vi "S4GUI.vi"() -> ()   [LabVIEW 2018] (continued)
                          tunnel: [w778 u32 13882323 u32 13882323] -> w773
                          tunnel: w775 -> [w777 _ _]
                          tunnel: w774 -> [w776 _ _]
                          frame Default {
                            n286 = case shown="True" w777 {
                              tunnel: [w779 w783] -> w778
                              tunnel: w776 -> [w779 w780]
                              frame False {
                              }
                              frame True {
                                n287 = Equal?(x=w780, y=u32 16776002) -> (x = y?=w782:bool)
                                n288 = case shown="False" w782 {
                                tunnel: [u32 16776002 u32 9346816] -> w783
                                frame False {
                                }
                                frame True {
                                }
                                }
                              }
                            }
                          }
                          frame "IDLE" {
                          }
                          frame "" {
                            # "sem resposta do ACS"
                          }
                        }
                      }
                    }
                    "Acq status string ch1" <- w701
                    n289 = case shown="True" w696 {
                      tunnel: w709 -> [_ w736]
                      tunnel: [u32 16739417 w738] -> w708
                      tunnel: w704 -> [_ w737]
                      tunnel: ["" ("CamStatus") w736] -> w698
                      frame False {
                      }
                      frame True {
                        n290 = property on="Acq status string ch3" class="Str"() -> ("Text.BGColor"=w739:u32)  [unwired: 2 in, 2 out]
                        n291 = case shown="Default" w736 {
                          tunnel: [w742 u32 13882323 u32 13882323] -> w738
                          tunnel: w737 -> [w741 _ _]
                          tunnel: w739 -> [w740 _ _]
                          frame Default {
                            n292 = case shown="True" w741 {
                              tunnel: [w743 w747] -> w742
                              tunnel: w740 -> [w743 w744]
                              frame False {
                              }
                              frame True {
                                n293 = Equal?(x=w744, y=u32 16776002) -> (x = y?=w746:bool)
                                n294 = case shown="True" w746 {
                                tunnel: [u32 16776002 u32 9346816] -> w747
                                frame False {
                                }
                                frame True {
                                }
                                }
                              }
                            }
                          }
                          frame "IDLE" {
                          }
                          frame "" {
                            # "sem resposta do ACS"
                          }
                        }
                      }
                    }
                    "Acq status string ch3" <- w698
                    n295 = case shown="True" w700 {
                      tunnel: w707 -> [_ w754]
                      tunnel: [u32 16739417 w756] -> w706
                      tunnel: w704 -> [_ w755]
                      tunnel: ["" ("CamStatus") w754] -> w699
                      frame False {
                      }
                      frame True {
                        n296 = property on="Acq status string ch2" class="Str"() -> ("Text.BGColor"=w757:u32)  [unwired: 2 in, 2 out]
                        n297 = case shown="\"IDLE\"" w754 {
                          tunnel: [w760 u32 13882323 u32 13882323] -> w756
                          tunnel: w755 -> [w759 _ _]
                          tunnel: w757 -> [w758 _ _]
                          frame Default {
                            n298 = case shown="False" w759 {
                              tunnel: [w761 w765] -> w760
                              tunnel: w758 -> [w761 w762]
                              frame False {
                              }
                              frame True {
                                n299 = Equal?(x=w762, y=u32 16776002) -> (x = y?=w764:bool)
                                n300 = case shown="True" w764 {
                                tunnel: [u32 16776002 u32 9346816] -> w765
                                frame False {
                                }
                                frame True {
                                }
                                }
                              }
                            }
                          }
                          frame "IDLE" {
                          }
                          frame "" {
                            # "sem resposta do ACS"
                          }
                        }
                      }
                    }
                    "Acq status string ch2" <- w699
                    n301 = property on="Acq status string ch2" class="Str"("Text.BGColor"=w706) -> ()  [unwired: 2 in, 2 out]
                    n302 = property on="Acq status string ch1" class="Str"("Text.BGColor"=w703) -> ()  [unwired: 2 in, 2 out]
                    n303 = property on="Acq status string ch3" class="Str"("Text.BGColor"=w708) -> ()  [unwired: 2 in, 2 out]
                    n304 = property on="Acq status string ch4" class="Str"("Text.BGColor"=w711) -> ()  [unwired: 2 in, 2 out]
                  }
                  frame #3 {
                    # "Atualiza status CANAL 1"
                    n305 = Unbundle By Name(w791) -> ("Frames done"=→"Exposure Done ch1":u32, "connection"=→"Channel 1" →"setupCH1":bool, "conf runing"=w788:bool)
                    n306 = property on="setupCH1" class="Bool (strict)"("Blinking"=w788) -> ()  [unwired: 2 in, 2 out]
                  }
                  frame #4 {
                    # "Atualiza status CANAL 2"
                    n307 = Unbundle By Name(w794) -> ("Frames done"=→"Exposure Done ch2":u32, "connection"=→"Channel 2" →"setupCH2":bool, "conf runing"=w792:bool)
                    n308 = property on="setupCH2" class="Bool (strict)"("Blinking"=w792) -> ()  [unwired: 2 in, 2 out]
                  }
                  frame #5 {
                    # "Atualiza status CANAL3"
                    n309 = Unbundle By Name(w798) -> ("Frames done"=→"Exposure Done ch3":u32, "connection"=→"Channel 3" →"setupCH3":bool, "conf runing"=w797:bool)
                    n310 = property on="setupCH3" class="Bool (strict)"("Blinking"=w797) -> ()  [unwired: 2 in, 2 out]
                  }
                  frame #6 {
                    # "Atualiza status CANAL4"
                    n311 = Unbundle By Name(w802) -> ("Frames done"=→"Exposure Done ch4":u32, "connection"=→"Channel 4" →"setupCH4":bool, "conf runing"=w801:bool)
                    n312 = property on="setupCH4" class="Bool (strict)"("Blinking"=w801) -> ()  [unwired: 2 in, 2 out]
                  }
                }
              }
              frame #9 {
                n313 = Unbundle By Name(w805) -> ("Instrument Status.mode"=w804:bool)
                n314 = case shown="True" w804 {
                  tunnel: [0 ("t") w819] -> w806
                  tunnel: w805 -> [_ w808]
                  frame False {
                    # "Fotometria: #PSD = 0"
                  }
                  frame True {
                    # "Polarimetria: calcula #PSD"
                    n315 = Unbundle By Name(w808) -> ("WPROT seq"=w812:u16)
                    n316 = Number To Boolean Array(number=w812) -> (Boolean array=w811:bool[])
                    n317 = for {
                      shift-right: [w823] -> w814
                      shift-left: 0 -> [w821]
                      tunnel: w811 -> [w820] mode=indexing
                      # "calcula qtd de 1s"
                      n318 = Increment(x=w821) -> (x+1=w822:i32)
                      n319 = Select(t=w822, s=w820, f=w821) -> (s? t:f=w823:i32)
                    }
                    n320 = property on="#Polarimetric Sequence Done" class="Slide (strict)"() -> ("Scale.Maximum"=w813:dbl)  [unwired: 2 in, 2 out]
                    n321 = To Long Integer(number=w813) -> (32bit integer=w815:i32)
                    n322 = Subtract(x=w815, y=w814) -> (x-y=w816:i32)
                    n323 = Decrement(x=w816) -> (x-1=w818:i32)
                    n324 = Less Than 0?(x=w818) -> (x < 0?=w817:bool)
                    n325 = Select(t=0, s=w817, f=w818) -> (s? t:f=w819:i32)
                  }
                }
                "#Polarimetric Sequence Done" <- w806
              }
              frame #10 {
                # "OVJ 2022-12-12: \nA visibilidade do Tab ObsEng sermpre \nacompanha a habilitação do tab4."
                n326 = Unbundle By Name(w828) -> ("Cluster ExpMode.tab4"=w825:T7, "Cluster Polarimetry"=w849:T15, "Cluster Mode Sync"=w859:T16)
                n327 = case shown="\"Disabled and Grayed Out\"" w825 {
                  tunnel: [TRUE ("Tabs Visible?") w861] -> w827
                  frame "Enabled", Default {
                  }
                  frame "Disabled and Grayed Out" {
                    n328 = disable-structure shown="Enabled" {
                      disable-tunnel: [TRUE ("Tabs Visible?") FALSE ("Tabs Visible?")] -> w861
                      frame Disabled {
                        # "DEBUG"
                      }
                      frame Enabled {
                      }
                    }
                  }
                }
                n329 = property on="Tab ObsEng" class="TabCtl (strict)"("Tabs Visible?"=w827) -> ()  [unwired: 2 in, 2 out]
                n330 = property on="Tab Acq Type" class="TabCtl (strict)"("DisabledEnum"=w825) -> (error out=w826:errorcluster)  [unwired: 2 in, 1 out]
                n331 = Unbundle By Name(w859) -> ("Start SM Text"=w858:string, "Star SM"=w857:T7, "Pause SM"=w856:T7, "Stop SM"=w855:T7, "Abort SM"=w854:T7, "#Index Cycles"=w853:T7, "#Cycles"=w852:T7, "SSM"=w851:T7, "Set SM"=w850:T7)
                n332 = property on="Observer" class="Str"(error in=w826, "DisabledEnum"=w825) -> (error out=w824:errorcluster)  [unwired: 1 in, 1 out]
                n333 = property on="Start SM" class="Bool"("BoolText.Text"=w858) -> ()  [unwired: 2 in, 2 out]
                n334 = property on="set keywords" class="Bool"(error in=w824, "DisabledEnum"=w825) -> ()  [unwired: 1 in, 2 out]
                n335 = property on="Start SM" class="Bool"("DisabledEnum"=w857) -> ()  [unwired: 2 in, 2 out]
                n336 = property on="Stop SM" class="Bool"("DisabledEnum"=w855) -> ()  [unwired: 2 in, 2 out]
                n337 = property on="Set SM" class="Bool"("DisabledEnum"=w850) -> ()  [unwired: 2 in, 2 out]
                n338 = property on="Pause SM" class="Bool"("DisabledEnum"=w856) -> ()  [unwired: 2 in, 2 out]
                n339 = property on="# Index Cycles" class="DigNum (strict)"("DisabledEnum"=w853) -> ()  [unwired: 2 in, 2 out]
                n340 = property on="# Cycles" class="DigNum (strict)"("DisabledEnum"=w852) -> ()  [unwired: 2 in, 2 out]
                n341 = property on="Abort SM" class="Bool"("DisabledEnum"=w854) -> ()  [unwired: 2 in, 2 out]
                n342 = property on="SSM" class="Ring (strict)"("DisabledEnum"=w851) -> ()  [unwired: 2 in, 2 out]
                n343 = Unbundle By Name(w849) -> ("Lambda Selector"=w848:T7, "Calibrator Selector"=w847:T7, "Set Waveplate"=w846:T7, "Select Positions"=w845:T7, "P0"=w844:T7, "P8"=w843:T7, "P1"=w842:T7, "P9"=w841:T7, "P2"=w840:T7, "P10"=w839:T7, "P3"=w838:T7, "P11"=w837:T7, "P4"=w836:T7, "P12"=w835:T7, "P5"=w834:T7, "P13"=w833:T7, "P6"=w832:T7, "P14"=w831:T7, "P7"=w830:T7, "P15"=w829:T7)
                n344 = property on="P0" class="Bool (strict)"("DisabledEnum"=w844) -> ()  [unwired: 2 in, 2 out]
                n345 = property on="Lambda Selector" class="Ring (strict)"("DisabledEnum"=w848) -> ()  [unwired: 2 in, 2 out]
                n346 = property on="Calibrator Selector" class="Ring (strict)"("DisabledEnum"=w847) -> ()  [unwired: 2 in, 2 out]
                n347 = property on="Set Waveplate" class="Bool"("DisabledEnum"=w846) -> ()  [unwired: 2 in, 2 out]
                n348 = property on="P1" class="Bool (strict)"("DisabledEnum"=w842) -> ()  [unwired: 2 in, 2 out]
                n349 = property on="P2" class="Bool (strict)"("DisabledEnum"=w840) -> ()  [unwired: 2 in, 2 out]
                n350 = property on="P3" class="Bool (strict)"("DisabledEnum"=w838) -> ()  [unwired: 2 in, 2 out]
                n351 = property on="P4" class="Bool (strict)"("DisabledEnum"=w836) -> ()  [unwired: 2 in, 2 out]
                n352 = property on="P5" class="Bool (strict)"("DisabledEnum"=w834) -> ()  [unwired: 2 in, 2 out]
                n353 = property on="P6" class="Bool (strict)"("DisabledEnum"=w832) -> ()  [unwired: 2 in, 2 out]
                n354 = property on="P7" class="Bool (strict)"("DisabledEnum"=w830) -> ()  [unwired: 2 in, 2 out]
                n355 = property on="Select Positions" class="Ring (strict)"("DisabledEnum"=w845) -> ()  [unwired: 2 in, 2 out]
                n356 = property on="P8" class="Bool (strict)"("DisabledEnum"=w843) -> ()  [unwired: 2 in, 2 out]
                n357 = property on="P15" class="Bool (strict)"("DisabledEnum"=w829) -> ()  [unwired: 2 in, 2 out]
                n358 = property on="P9" class="Bool (strict)"("DisabledEnum"=w841) -> ()  [unwired: 2 in, 2 out]
                n359 = property on="P10" class="Bool (strict)"("DisabledEnum"=w839) -> ()  [unwired: 2 in, 2 out]
                n360 = property on="P11" class="Bool (strict)"("DisabledEnum"=w837) -> ()  [unwired: 2 in, 2 out]
                n361 = property on="P12" class="Bool (strict)"("DisabledEnum"=w835) -> ()  [unwired: 2 in, 2 out]
                n362 = property on="P13" class="Bool (strict)"("DisabledEnum"=w833) -> ()  [unwired: 2 in, 2 out]
                n363 = property on="P14" class="Bool (strict)"("DisabledEnum"=w831) -> ()  [unwired: 2 in, 2 out]
              }
              frame #11 {
                n364 = Unbundle By Name(w875) -> ("Cluster Mode CH1"=w874:T17)
                n365 = Unbundle By Name(w874) -> ("Start ch1 Text"=w873:string, "#cycles ch1"=w872:T7, "Start ch1"=w871:T7, "Pause ch1"=w870:T7, "Abort ch1"=w869:T7, "Stop ch1"=w868:T7, "Exptime ch1"=w867:T7, "Exp ch1"=w866:T7, "Set Cooler"=w865:T7, "Set Temp"=w864:T7)
                n366 = property on="Start ch1" class="Bool"("BoolText.Text"=w873) -> ()  [unwired: 2 in, 2 out]
                n367 = property on="Abort ch1" class="Bool"("DisabledEnum"=w869) -> ()  [unwired: 2 in, 2 out]
                n368 = property on="Stop ch1" class="Bool"("DisabledEnum"=w868) -> ()  [unwired: 2 in, 2 out]
                n369 = property on="#cycles ch1" class="DigNum (strict)"("DisabledEnum"=w872) -> ()  [unwired: 2 in, 2 out]
                n370 = property on="Cooler 1" class="Bool (strict)"("DisabledEnum"=w865) -> ()  [unwired: 2 in, 2 out]
                n371 = property on="Exptime ch1" class="DigNum (strict)"("DisabledEnum"=w867) -> ()  [unwired: 2 in, 2 out]
                n372 = property on="Start ch1" class="Bool"("DisabledEnum"=w871) -> ()  [unwired: 2 in, 2 out]
                n373 = property on="Set Temp 1" class="Bool"("DisabledEnum"=w864) -> ()  [unwired: 2 in, 2 out]
                n374 = property on="Exp ch1" class="DigNum (strict)"("DisabledEnum"=w866) -> ()  [unwired: 2 in, 2 out]
                n375 = property on="Pause ch1" class="Bool"("DisabledEnum"=w870) -> ()  [unwired: 2 in, 2 out]
              }
              frame #12 {
                n376 = Unbundle By Name(w887) -> ("Cluster Mode CH2"=w886:T18)
                n377 = Unbundle By Name(w886) -> ("Start ch2 Text"=w885:string, "#cycles ch2"=w884:T7, "Start ch2"=w883:T7, "Pause ch2"=w882:T7, "Stop ch2"=w881:T7, "Abort ch2"=w880:T7, "Exptime ch2"=w879:T7, "Exp ch2"=w878:T7, "Set Cooler"=w877:T7, "Set Temp"=w876:T7)
                n378 = property on="Start ch2" class="Bool"("BoolText.Text"=w885) -> ()  [unwired: 2 in, 2 out]
                n379 = property on="Stop ch2" class="Bool"("DisabledEnum"=w881) -> ()  [unwired: 2 in, 2 out]
                n380 = property on="Abort ch2" class="Bool"("DisabledEnum"=w880) -> ()  [unwired: 2 in, 2 out]
                n381 = property on="Cooler 2" class="Bool (strict)"("DisabledEnum"=w877) -> ()  [unwired: 2 in, 2 out]
                n382 = property on="#cycles ch2" class="DigNum (strict)"("DisabledEnum"=w884) -> ()  [unwired: 2 in, 2 out]
                n383 = property on="Exptime ch2" class="DigNum (strict)"("DisabledEnum"=w879) -> ()  [unwired: 2 in, 2 out]
                n384 = property on="Set Temp 2" class="Bool"("DisabledEnum"=w876) -> ()  [unwired: 2 in, 2 out]
                n385 = property on="Start ch2" class="Bool"("DisabledEnum"=w883) -> ()  [unwired: 2 in, 2 out]
                n386 = property on="Exp ch2" class="DigNum (strict)"("DisabledEnum"=w878) -> ()  [unwired: 2 in, 2 out]
                n387 = property on="Pause ch2" class="Bool"("DisabledEnum"=w882) -> ()  [unwired: 2 in, 2 out]
              }
              frame #13 {
                n388 = Unbundle By Name(w899) -> ("Cluster Mode CH3"=w898:T19)
                n389 = Unbundle By Name(w898) -> ("Start ch3 Text"=w897:string, "#cycles ch3"=w896:T7, "Start ch3"=w895:T7, "Pause ch3"=w894:T7, "Stop ch3"=w893:T7, "Abort ch3"=w892:T7, "Exptime ch3"=w891:T7, "Exp ch3"=w890:T7, "Set Cooler"=w889:T7, "Set Temp"=w888:T7)
                n390 = property on="Start ch3" class="Bool"("BoolText.Text"=w897) -> ()  [unwired: 2 in, 2 out]
                n391 = property on="Stop ch3" class="Bool"("DisabledEnum"=w893) -> ()  [unwired: 2 in, 2 out]
                n392 = property on="Abort ch3" class="Bool"("DisabledEnum"=w892) -> ()  [unwired: 2 in, 2 out]
                n393 = property on="Cooler 3" class="Bool (strict)"("DisabledEnum"=w889) -> ()  [unwired: 2 in, 2 out]
                n394 = property on="#cycles ch3" class="DigNum (strict)"("DisabledEnum"=w896) -> ()  [unwired: 2 in, 2 out]
                n395 = property on="Set Temp 3" class="Bool"("DisabledEnum"=w888) -> ()  [unwired: 2 in, 2 out]
                n396 = property on="Exptime ch3" class="DigNum (strict)"("DisabledEnum"=w891) -> ()  [unwired: 2 in, 2 out]
                n397 = property on="Start ch3" class="Bool"("DisabledEnum"=w895) -> ()  [unwired: 2 in, 2 out]
                n398 = property on="Exp ch3" class="DigNum (strict)"("DisabledEnum"=w890) -> ()  [unwired: 2 in, 2 out]
                n399 = property on="Pause ch3" class="Bool"("DisabledEnum"=w894) -> ()  [unwired: 2 in, 2 out]
              }
              frame #14 {
                n400 = Unbundle By Name(w911) -> ("Cluster Mode CH4"=w910:T20)
                n401 = Unbundle By Name(w910) -> ("Start ch4 Text"=w909:string, "#cycles ch4"=w908:T7, "Start ch4"=w907:T7, "Pause ch4"=w906:T7, "Stop ch4"=w905:T7, "Abort ch4"=w904:T7, "Exptime ch4"=w903:T7, "Exp ch4"=w902:T7, "Set Cooler"=w901:T7, "Set Temp"=w900:T7)
                n402 = property on="Start ch4" class="Bool"("BoolText.Text"=w909) -> ()  [unwired: 2 in, 2 out]
                n403 = property on="Stop ch4" class="Bool"("DisabledEnum"=w905) -> ()  [unwired: 2 in, 2 out]
                n404 = property on="Cooler 4" class="Bool (strict)"("DisabledEnum"=w901) -> ()  [unwired: 2 in, 2 out]
                n405 = property on="Set Temp 4" class="Bool"("DisabledEnum"=w900) -> ()  [unwired: 2 in, 2 out]
                n406 = property on="Abort ch4" class="Bool"("DisabledEnum"=w904) -> ()  [unwired: 2 in, 2 out]
                n407 = property on="#cycles ch4" class="DigNum (strict)"("DisabledEnum"=w908) -> ()  [unwired: 2 in, 2 out]
                n408 = property on="Exptime ch4" class="DigNum (strict)"("DisabledEnum"=w903) -> ()  [unwired: 2 in, 2 out]
                n409 = property on="Start ch4" class="Bool"("DisabledEnum"=w907) -> ()  [unwired: 2 in, 2 out]
                n410 = property on="Exp ch4" class="DigNum (strict)"("DisabledEnum"=w902) -> ()  [unwired: 2 in, 2 out]
                n411 = property on="Pause ch4" class="Bool"("DisabledEnum"=w906) -> ()  [unwired: 2 in, 2 out]
              }
              frame #15 {
                # "Carrega coluna do Channel 1"
                # "Aba:  Eng->Camera"
                n412 = Unbundle By Name(w995) -> ("ChannelA_CCD"=w919:T21, "CHA_Checked Params"=w986:T22, "ChannelA_Status.connection"=w918:bool)
                n413 = Unbundle By Name(w986) -> ("ACQUISITION_MODE"=w943:bool, "TRIGGER_MODE"=w944:bool, "READ_MODE"=w945:bool, "PREAMP"=w953:bool, "READOUT_RATE"=w954:bool, "VERTICAL_SHIFT_SPEED"=w955:bool, "EM_MODE"=w956:bool, "EM_GAIN"=w946:bool, "SHUTTER_MODE"=w947:bool, "SHUTTER_TTL"=w948:bool, "SHUTTER_OPENING_TIME"=w949:bool, "SHUTTER_CLOSING_TIME"=w950:bool, "VBIN"=w951:bool, "HBIN"=w952:bool, "INITIAL_LINE"=w964:bool, "INITIAL_COLUMN"=w980:bool, "FINAL_LINE"=w985:bool, "FINAL_COLUMN"=w978:bool, "FRAME_TRANSFER"=w974:bool, "VERTICAL_CLOCK_VOLTAGE"=w973:bool, "AD_CHANNEL"=w972:bool)
                n414 = Unbundle By Name(w919) -> ("INITIAL_LINE"=w941:u16, "INITIAL_COLUMN"=w940:u16, "FINAL_LINE"=w939:u16, "FINAL_COLUMN"=w938:u16, "VBIN"=w937:u16, "HBIN"=w936:u16, "PREAMP"=w935:u8, "EM_GAIN"=w934:u16, "READOUT_RATE"=w933:u8, "SHUTTER_OPENNING_TIME"=w932:u16, "SHUTTER_CLOSING_TIME"=w931:u16, "VERTICAL_SHIFT_SPEED"=w930:u8, "READ_MODE"=w929:u8, "VERTICAL_CLOCK_VOLTAGE"=w928:u8, "AD_CHANNEL"=w927:u32, "SHUTTER_MODE"=w926:u8, "SHUTTER_TTL"=w925:u8, "TRIGGER_MODE"=w924:u8, "FRAME_TRANSFER"=w923:bool, "ACQUISITION_MODE"=w921:u8, "EM_MODE"=w920:u8)
                n415 = Equal?(x=w990, y="none") -> (x = y?=w987:bool)
                n416 = Equal?(x=w990, y="default.cfg") -> (x = y?=w988:bool)
                n417 = Or(x=w988, y=w987) -> (x .or. y?=w989:bool)
                n418 = case shown="True" w989 {
                  tunnel: [T7."Enabled" ("Disabled") T7."Disabled and Grayed Out" ("Disabled")] -> w992
                  frame False {
                    # "Se Curr Conf File != default.cfg,\nhabilita botão de Salvar."
                  }
                  frame True {
                    # "Não é permitido salvar em \ncima de default.cfg"
                  }
                }
                n419 = case shown="True" w918 {
                  tunnel: w919 -> [_ w1003]
                  tunnel: [w996 w1002] -> w917
                  tunnel: [w996 w1001] -> w916
                  tunnel: [w996 w1000] -> w915
                  tunnel: [w996 w999] -> w914
                  tunnel: [w996 w998] -> w913
                  tunnel: [w996 w997] -> w912
                  frame False {
                    w996 = "" ("RO1")
                  }
                  frame True {
                    n420 = stacked-sequence "Atualizacao dos indicadores inferiores do CANAL A da tela principal" {
                      tunnel: w1003 -> [w1018 w1021 w1026 w1035 w1038 w1042]
                      tunnel: [w1004 _ _ _ _ _] -> w1002
                      tunnel: [_ w1019 _ _ _ _] -> w1001
                      tunnel: [_ _ w1024 _ _ _] -> w1000
                      tunnel: [_ _ _ w1029 _ _] -> w999
                      tunnel: [_ _ _ _ w1036 _] -> w998
                      tunnel: [_ _ _ _ _ w1039] -> w997
                      frame #0 {
                        # "SubImage"
                        n421 = Unbundle By Name(w1018) -> ("INITIAL_LINE"=w1016:u16, "FINAL_LINE"=w1015:u16, "INITIAL_COLUMN"=w1014:u16, "FINAL_COLUMN"=w1013:u16)
                        n422 = Number To Decimal String(number=w1016) -> (decimal integer string=w1012:string)  [unwired: 1 in]
                        n423 = Number To Decimal String(number=w1015) -> (decimal integer string=w1010:string)  [unwired: 1 in]
                        n424 = Number To Decimal String(number=w1014) -> (decimal integer string=w1008:string)  [unwired: 1 in]
                        n425 = Number To Decimal String(number=w1013) -> (decimal integer string=w1006:string)  [unwired: 1 in]
                        n426 = Concatenate Strings("[", w1012, ":", w1010, ",", w1008, ":", w1006, "]") -> (w1004:string)
                      }
                      frame #1 {
                        # "Em Active"
                        n427 = Unbundle By Name(w1021) -> ("EM_MODE"=w1020:u8)
                        n428 = case shown="0, Default" w1020 {
                          tunnel: ["Electron M." ("EmActive1") "Convent." ("EmActive1")] -> w1019
                          frame 0, Default {
                          }
                          frame 1 {
                          }
                        }
                      }
                      frame #2 {
                        # "Pre Amp"
                        n429 = Unbundle By Name(w1026) -> ("PREAMP"=w1025:u8)
                        n430 = case shown="1" w1025 {
                          tunnel: ["Gain 1" ("EmActive1") "Gain 2" ("EmActive1")] -> w1024
                          frame 0, Default {
                          }
                          frame 1 {
                          }
                        }
                      }
                      frame #3 {
                        # "Binning"
                        n431 = Unbundle By Name(w1035) -> ("VBIN"=w1034:u16, "HBIN"=w1033:u16)
                        n432 = Number To Decimal String(number=w1033) -> (decimal integer string=w1030:string)  [unwired: 1 in]
                        n433 = Number To Decimal String(number=w1034) -> (decimal integer string=w1032:string)  [unwired: 1 in]
                        n434 = Concatenate Strings(w1032, "x", w1030) -> (w1029:string)
                      }
                      frame #4 {
                        # "Gain"
                        n435 = Unbundle By Name(w1038) -> ("EM_GAIN"=w1037:u16)
                        n436 = Number To Decimal String(number=w1037) -> (decimal integer string=w1036:string)  [unwired: 1 in]
                      }
                      frame #5 {
                        # "Readout"
                        n437 = Unbundle By Name(w1042) -> ("EM_MODE"=w1041:u8, "READOUT_RATE"=w1040:u8)
                        n438 = case shown="1" w1041 {
                          tunnel: w1040 -> [w1044 w1050]
                          tunnel: [w1043 w1049] -> w1039
                          frame 0, Default {
                            n439 = case shown="3" w1044 {
                              tunnel: ["30 MHz" ("EmActive1") "20 MHz" ("EmActive1") "10 MHz" ("EmActive1") "1 MHz" ("EmActive1")] -> w1043
                              frame 0, Default {
                              }
                              frame 1 {
                              }
                              frame 2 {
                              }
                              frame 3 {
                              }
                            }
                          }
                          frame 1 {
                            n440 = case shown="1" w1050 {
                              tunnel: ["1 MHz" ("EmActive1") "0.1 MHz" ("EmActive1")] -> w1049
                              frame 0, Default {
                              }
                              frame 1 {
                              }
                            }
                          }
                        }
                      }
                    }
                  }
                }
                n441 = Not(x=w978) -> (.not. x?=w979:bool)
                n442 = Not(x=w974) -> (.not. x?=w976:bool)
                n443 = Not(x=w973) -> (.not. x?=w977:bool)
                n444 = Not(x=w972) -> (.not. x?=w975:bool)
                n445 = Not(x=w964) -> (.not. x?=w982:bool)
                n446 = Not(x=w980) -> (.not. x?=w981:bool)
                n447 = Not(x=w985) -> (.not. x?=w984:bool)
                n448 = property on="Image FInal Column" class="DigNum (strict)"("Blinking"=w979) -> ()  [unwired: 2 in, 2 out]
                n449 = property on="Frame Transfer" class="Bool (strict)"("Blinking"=w976) -> ()  [unwired: 2 in, 2 out]
                n450 = property on="Vertical Clock Voltage" class="Ring (strict)"("Blinking"=w977) -> ()  [unwired: 2 in, 2 out]
                n451 = property on="A/D  Channel" class="DigNum (strict)"("Blinking"=w975) -> ()  [unwired: 2 in, 2 out]
                n452 = property on="Image Initial Line" class="DigNum (strict)"("Blinking"=w982) -> ()  [unwired: 2 in, 2 out]
                n453 = property on="Image Initial Column" class="DigNum (strict)"("Blinking"=w981) -> ()  [unwired: 2 in, 2 out]
                n454 = property on="Image Final Line" class="DigNum (strict)"("Blinking"=w984) -> ()  [unwired: 2 in, 2 out]
                n455 = property on="Save Button" class="Bool (strict)"("DisabledEnum"=w992) -> ()  [unwired: 2 in, 2 out]
                n456 = Not(x=w949) -> (.not. x?=w968:bool)
                n457 = Not(x=w950) -> (.not. x?=w970:bool)
                n458 = Not(x=w951) -> (.not. x?=w969:bool)
                n459 = Not(x=w952) -> (.not. x?=w971:bool)
                n460 = Not(x=w946) -> (.not. x?=w966:bool)
                n461 = Not(x=w947) -> (.not. x?=w967:bool)
                n462 = Not(x=w948) -> (.not. x?=w965:bool)
                n463 = property on="Shutter Openning Time" class="DigNum (strict)"("Blinking"=w968) -> ()  [unwired: 2 in, 2 out]
                n464 = property on="Shutter Closing Time" class="DigNum (strict)"("Blinking"=w970) -> ()  [unwired: 2 in, 2 out]
                n465 = property on="Vertical Binning" class="DigNum (strict)"("Blinking"=w969) -> ()  [unwired: 2 in, 2 out]
                n466 = property on="Horizontal Binning" class="DigNum (strict)"("Blinking"=w971) -> ()  [unwired: 2 in, 2 out]
                n467 = property on="CCD EM Gain" class="DigNum (strict)"("Blinking"=w966) -> ()  [unwired: 2 in, 2 out]
                n468 = property on="Shutter Mode" class="Ring (strict)"("Blinking"=w967) -> ()  [unwired: 2 in, 2 out]
                n469 = property on="Shutter TTL" class="Ring (strict)"("Blinking"=w965) -> ()  [unwired: 2 in, 2 out]
                n470 = First Call?() -> (First Call?: T/F=w942:bool)
                n471 = case shown="True" w942 {
                  tunnel: w941 -> [_ w1073]
                  tunnel: w940 -> [_ w1072]
                  tunnel: w939 -> [_ w1071]
                  tunnel: w938 -> [_ w1070]
                  tunnel: w937 -> [_ w1069]
                  tunnel: w936 -> [_ w1068]
                  tunnel: w935 -> [_ w1067]
                  tunnel: w934 -> [_ w1066]
                  tunnel: w933 -> [_ w1065]
                  tunnel: w932 -> [_ w1064]
                  tunnel: w931 -> [_ w1063]
                  tunnel: w930 -> [_ w1062]
                  tunnel: w929 -> [_ w1061]
                  tunnel: w928 -> [_ w1060]
                  tunnel: w927 -> [_ w1059]
                  tunnel: w926 -> [_ w1058]
                  tunnel: w925 -> [_ w1057]
                  tunnel: w924 -> [_ w1056]
                  tunnel: w923 -> [_ w1055]
                  tunnel: w921 -> [_ w1054]
                  tunnel: w920 -> [_ w1053]
                  frame False {
                  }
                  frame True {
                    n472 = local read "Input Cluster"() -> (w1077:T5)
                    n473 = Unbundle By Name(w1077) -> ("Parameters"=w1075:T23)
                    n474 = Bundle By Name(cluster=w1075, "Image \nInitial Line"=w1073, "Image\nInitial Column"=w1072, "Image\nFinal Line"=w1071, "Image\nFInal Column"=w1070, "Vertical\nBinning"=w1069, "Horizontal\nBinning"=w1068, "Pre-amplification\nGain"=w1067, "CCD\nEM Gain"=w1066, "Readout\nRate"=w1065, "Shutter\nOpenning Time"=w1064, "Shutter\nClosing Time"=w1063, "Vertical\nShift Speed"=w1062, "Read\nMode"=w1061, "Vertical\nClock Voltage"=w1060, "A/D \nChannel"=w1059, "Shutter\nMode"=w1058, "Shutter\nTTL"=w1057, "Trigger\nMode"=w1056, "Frame\nTransfer"=w1055, "Acquisition\nMode"=w1054, "CCD \nEM Mode"=w1053) -> (w1074:T23)
                    n475 = Bundle By Name(cluster=w1077, "Parameters"=w1074) -> (w1076:T5)
                    n476 = local write "Input Cluster"(w1076) -> ()
                  }
                }
                n477 = Not(x=w943) -> (.not. x?=w957:bool)
                n478 = local read "Cameras Cluster"() -> (w994:T6)
                n479 = Bundle By Name(cluster=w994, "Current Configuration.Image Initial Line"=w941, "Current Configuration.Image Initial Column"=w940, "Current Configuration.Image Final Line"=w939, "Current Configuration.Image FInal Column"=w938, "Current Configuration.Vertical Binning"=w937, "Current Configuration.Horizontal Binning"=w936, "Current Configuration.Pre-amplification Gain"=w935, "Current Configuration.CCD EM Gain"=w934, "Current Configuration.Readout Rate"=w933, "Current Configuration.Shutter Openning Time"=w932, "Current Configuration.Shutter Closing Time"=w931, "Current Configuration.Vertical Shift Speed"=w930, "Current Configuration.Read Mode"=w929, "Current Configuration.Vertical Clock Voltage"=w928, "Current Configuration.A/D  Channel"=w927, "Current Configuration.Shutter Mode"=w926, "Current Configuration.Shutter TTL"=w925, "Current Configuration.Trigger Mode"=w924, "Current Configuration.Frame Transfer"=w923, "Current Configuration.Acquisition Mode"=w921, "Current Configuration.CCD EM Mode"=w920) -> (w922:T6)
                n480 = Not(x=w954) -> (.not. x?=w960:bool)
                n481 = Not(x=w955) -> (.not. x?=w958:bool)
                n482 = Not(x=w956) -> (.not. x?=w959:bool)
                n483 = Not(x=w944) -> (.not. x?=w962:bool)
                n484 = Not(x=w945) -> (.not. x?=w961:bool)
                n485 = Not(x=w953) -> (.not. x?=w963:bool)
                n486 = local write "RO1"(w912) -> ()
                n487 = local write "SI1"(w917) -> ()
                n488 = local write "EA1"(w916) -> ()
                n489 = local write "PA1"(w915) -> ()
                n490 = local write "B1"(w914) -> ()
                n491 = local write "G1"(w913) -> ()
                n492 = property on="Acquisition Mode" class="Ring (strict)"("Blinking"=w957) -> ()  [unwired: 2 in, 2 out]
                n493 = property on="Readout Rate" class="Ring (strict)"("Blinking"=w960) -> ()  [unwired: 2 in, 2 out]
                n494 = property on="Vertical Shift Speed" class="Ring (strict)"("Blinking"=w958) -> ()  [unwired: 2 in, 2 out]
                n495 = property on="CCD EM Mode" class="Ring (strict)"("Blinking"=w959) -> ()  [unwired: 2 in, 2 out]
                n496 = property on="Trigger Mode" class="Ring (strict)"("Blinking"=w962) -> ()  [unwired: 2 in, 2 out]
                n497 = property on="Read Mode" class="Ring (strict)"("Blinking"=w961) -> ()  [unwired: 2 in, 2 out]
                n498 = property on="Pre-amplification Gain" class="Ring (strict)"("Blinking"=w963) -> ()  [unwired: 2 in, 2 out]
                n499 = local write "Cameras Cluster"(w922) -> ()
                n500 = Compound Arithmetic op=AND(w943, w944, w945, w953, w954, w955, w956, w946, w947, w948, w949, w950, w951, w952, w964, w980, w985, w978, w974, w973, w972) -> (→"CCD checked 1":bool)
                "Current Configuration File:" <- w990
              }
              frame #16 {
                # "Carrega coluna do Channel 2"
                # "Aba:  Eng->Camera"
                n501 = Unbundle By Name(w1155) -> ("ChannelB_CCD"=w1087:T21, "CHB_Checked Params"=w1088:T22, "ChannelB_Status.connection"=w1086:bool)
                n502 = Unbundle By Name(w1088) -> ("ACQUISITION_MODE"=w1106:bool, "TRIGGER_MODE"=w1105:bool, "READ_MODE"=w1104:bool, "PREAMP"=w1103:bool, "READOUT_RATE"=w1102:bool, "VERTICAL_SHIFT_SPEED"=w1101:bool, "EM_MODE"=w1100:bool, "EM_GAIN"=w1113:bool, "SHUTTER_MODE"=w1112:bool, "SHUTTER_TTL"=w1111:bool, "SHUTTER_OPENING_TIME"=w1110:bool, "SHUTTER_CLOSING_TIME"=w1109:bool, "VBIN"=w1108:bool, "HBIN"=w1107:bool, "INITIAL_LINE"=w1120:bool, "INITIAL_COLUMN"=w1119:bool, "FINAL_LINE"=w1118:bool, "FINAL_COLUMN"=w1117:bool, "FRAME_TRANSFER"=w1116:bool, "VERTICAL_CLOCK_VOLTAGE"=w1115:bool, "AD_CHANNEL"=w1114:bool)
                n503 = case shown="True" w1086 {
                  tunnel: w1087 -> [_ w1163]
                  tunnel: [w1156 w1162] -> w1085
                  tunnel: [w1156 w1161] -> w1084
                  tunnel: [w1156 w1160] -> w1083
                  tunnel: [w1156 w1159] -> w1082
                  tunnel: [w1156 w1158] -> w1081
                  tunnel: [w1156 w1157] -> w1080
                  frame False {
                    w1156 = "" ("EmActive1")
                  }
                  frame True {
                    n504 = stacked-sequence "Atualizacao dos indicadores inferiores do CANAL B da tela principal" {
                      tunnel: w1163 -> [w1178 w1181 w1186 w1195 w1198 w1202]
                      tunnel: [_ w1179 _ _ _ _] -> w1162
                      tunnel: [_ _ w1184 _ _ _] -> w1161
                      tunnel: [_ _ _ w1189 _ _] -> w1160
                      tunnel: [_ _ _ _ w1196 _] -> w1159
                      tunnel: [_ _ _ _ _ w1199] -> w1158
                      tunnel: [w1164 _ _ _ _ _] -> w1157
                      frame #0 {
                        # "SubImage"
                        n505 = Unbundle By Name(w1178) -> ("INITIAL_LINE"=w1176:u16, "FINAL_LINE"=w1175:u16, "INITIAL_COLUMN"=w1174:u16, "FINAL_COLUMN"=w1173:u16)
                        n506 = Number To Decimal String(number=w1176) -> (decimal integer string=w1172:string)  [unwired: 1 in]
                        n507 = Number To Decimal String(number=w1175) -> (decimal integer string=w1170:string)  [unwired: 1 in]
                        n508 = Number To Decimal String(number=w1174) -> (decimal integer string=w1168:string)  [unwired: 1 in]
                        n509 = Number To Decimal String(number=w1173) -> (decimal integer string=w1166:string)  [unwired: 1 in]
                        n510 = Concatenate Strings("[", w1172, ":", w1170, ",", w1168, ":", w1166, "]") -> (w1164:string)
                      }
                      frame #1 {
                        # "Em Active"
                        n511 = Unbundle By Name(w1181) -> ("EM_MODE"=w1180:u8)
                        n512 = case shown="0, Default" w1180 {
                          tunnel: ["Electron M." ("EmActive1") "Convent." ("EmActive1")] -> w1179
                          frame 0, Default {
                          }
                          frame 1 {
                          }
                        }
                      }
                      frame #2 {
                        # "Pre Amp"
                        n513 = Unbundle By Name(w1186) -> ("PREAMP"=w1185:u8)
                        n514 = case shown="1" w1185 {
                          tunnel: ["Gain 1" ("EmActive1") "Gain 2" ("EmActive1")] -> w1184
                          frame 0, Default {
                          }
                          frame 1 {
                          }
                        }
                      }
                      frame #3 {
                        # "Binning"
                        n515 = Unbundle By Name(w1195) -> ("VBIN"=w1194:u16, "HBIN"=w1193:u16)
                        n516 = Number To Decimal String(number=w1193) -> (decimal integer string=w1191:string)  [unwired: 1 in]
                        n517 = Number To Decimal String(number=w1194) -> (decimal integer string=w1192:string)  [unwired: 1 in]
                        n518 = Concatenate Strings(w1192, "x", w1191) -> (w1189:string)
                      }
                      frame #4 {
                        # "Gain"
                        n519 = Unbundle By Name(w1198) -> ("EM_GAIN"=w1197:u16)
                        n520 = Number To Decimal String(number=w1197) -> (decimal integer string=w1196:string)  [unwired: 1 in]
                      }
                      frame #5 {
                        # "Readout"
                        n521 = Unbundle By Name(w1202) -> ("EM_MODE"=w1201:u8, "READOUT_RATE"=w1200:u8)
                        n522 = case shown="0, Default" w1201 {
                          tunnel: w1200 -> [w1204 w1210]
                          tunnel: [w1203 w1209] -> w1199
                          frame 0, Default {
                            n523 = case shown="0, Default" w1204 {
                              tunnel: ["30 MHz" ("EmActive1") "20 MHz" ("EmActive1") "10 MHz" ("EmActive1") "1 MHz" ("EmActive1")] -> w1203
                              frame 0, Default {
                              }
                              frame 1 {
                              }
                              frame 2 {
                              }
                              frame 3 {
                              }
                            }
                          }
                          frame 1 {
                            n524 = case shown="1" w1210 {
                              tunnel: ["1 MHz" ("EmActive1") "0.1 MHz" ("EmActive1")] -> w1209
                              frame 0, Default {
                              }
                              frame 1 {
                              }
                            }
                          }
                        }
                      }
                    }
                  }
                }
                n525 = Unbundle By Name(w1087) -> ("INITIAL_LINE"=w1093:u16, "INITIAL_COLUMN"=w1091:u16, "FINAL_LINE"=w1094:u16, "FINAL_COLUMN"=w1092:u16, "VBIN"=w1097:u16, "HBIN"=w1152:u16, "PREAMP"=w1096:u8, "EM_GAIN"=w1095:u16, "READOUT_RATE"=w1090:u8, "SHUTTER_OPENNING_TIME"=w1151:u16, "SHUTTER_CLOSING_TIME"=w1150:u16, "VERTICAL_SHIFT_SPEED"=w1149:u8, "READ_MODE"=w1148:u8, "VERTICAL_CLOCK_VOLTAGE"=w1147:u8, "AD_CHANNEL"=w1146:u32, "SHUTTER_MODE"=w1143:u8, "SHUTTER_TTL"=w1144:u8, "TRIGGER_MODE"=w1098:u8, "FRAME_TRANSFER"=w1099:bool, "ACQUISITION_MODE"=w1145:u8, "EM_MODE"=w1089:u8)
                n526 = Not(x=w1117) -> (.not. x?=w1138:bool)
                n527 = Not(x=w1116) -> (.not. x?=w1136:bool)
                n528 = Not(x=w1115) -> (.not. x?=w1137:bool)
                n529 = Not(x=w1114) -> (.not. x?=w1135:bool)
                n530 = Not(x=w1120) -> (.not. x?=w1140:bool)
                n531 = Not(x=w1119) -> (.not. x?=w1139:bool)
                n532 = Not(x=w1118) -> (.not. x?=w1141:bool)
                n533 = property on="Image FInal Column 2" class="DigNum (strict)"("Blinking"=w1138) -> ()  [unwired: 2 in, 2 out]
                n534 = property on="Frame Transfer 2" class="Bool (strict)"("Blinking"=w1136) -> ()  [unwired: 2 in, 2 out]
                n535 = property on="Vertical Clock Voltage 2" class="Ring (strict)"("Blinking"=w1137) -> ()  [unwired: 2 in, 2 out]
                n536 = property on="A/D Channel 2" class="DigNum (strict)"("Blinking"=w1135) -> ()  [unwired: 2 in, 2 out]
                n537 = property on="Image Initial Line 2" class="DigNum (strict)"("Blinking"=w1140) -> ()  [unwired: 2 in, 2 out]
                n538 = property on="Image Initial Column 2" class="DigNum (strict)"("Blinking"=w1139) -> ()  [unwired: 2 in, 2 out]
                n539 = property on="Image Final Line 2" class="DigNum (strict)"("Blinking"=w1141) -> ()  [unwired: 2 in, 2 out]
                n540 = Not(x=w1110) -> (.not. x?=w1131:bool)
                n541 = Not(x=w1109) -> (.not. x?=w1133:bool)
                n542 = Not(x=w1108) -> (.not. x?=w1132:bool)
                n543 = Not(x=w1107) -> (.not. x?=w1134:bool)
                n544 = Not(x=w1113) -> (.not. x?=w1129:bool)
                n545 = Not(x=w1112) -> (.not. x?=w1130:bool)
                n546 = Not(x=w1111) -> (.not. x?=w1128:bool)
                n547 = property on="Shutter Openning Time 2" class="DigNum (strict)"("Blinking"=w1131) -> ()  [unwired: 2 in, 2 out]
                n548 = property on="Shutter Closing Time 2" class="DigNum (strict)"("Blinking"=w1133) -> ()  [unwired: 2 in, 2 out]
                n549 = property on="Vertical Binning 2" class="DigNum (strict)"("Blinking"=w1132) -> ()  [unwired: 2 in, 2 out]
                n550 = property on="Horizontal Binning 2" class="DigNum (strict)"("Blinking"=w1134) -> ()  [unwired: 2 in, 2 out]
                n551 = property on="CCD EM Gain 2" class="DigNum (strict)"("Blinking"=w1129) -> ()  [unwired: 2 in, 2 out]
                n552 = property on="Shutter Mode 2" class="Ring (strict)"("Blinking"=w1130) -> ()  [unwired: 2 in, 2 out]
                n553 = property on="Shutter TTL 2" class="Ring (strict)"("Blinking"=w1128) -> ()  [unwired: 2 in, 2 out]
                n554 = local read "Cameras Cluster"() -> (w1154:T6)
                n555 = Bundle By Name(cluster=w1154, "Current Configuration.Image Initial Line 2"=w1093, "Current Configuration.Image Initial Column 2"=w1091, "Current Configuration.Image Final Line 2"=w1094, "Current Configuration.Image FInal Column 2"=w1092, "Current Configuration.Vertical Binning 2"=w1097, "Current Configuration.Horizontal Binning 2"=w1152, "Current Configuration.Pre-amplification Gain 2"=w1096, "Current Configuration.CCD EM Gain 2"=w1095, "Current Configuration.Readout Rate 2"=w1090, "Current Configuration.Shutter Openning Time 2"=w1151, "Current Configuration.Shutter Closing Time 2"=w1150, "Current Configuration.Vertical Shift Speed 2"=w1149, "Current Configuration.Read Mode 2"=w1148, "Current Configuration.Vertical Clock Voltage 2"=w1147, "Current Configuration.A/D Channel 2"=w1146, "Current Configuration.Shutter Mode 2"=w1143, "Current Configuration.Shutter TTL 2"=w1144, "Current Configuration.Trigger Mode 2"=w1098, "Current Configuration.Frame Transfer 2"=w1099, "Current Configuration.Acquisition Mode 2"=w1145, "Current Configuration.CCD EM Mode 2"=w1089) -> (w1153:T6)
                n556 = local write "PA2"(w1084) -> ()
                n557 = local write "B2"(w1083) -> ()
                n558 = local write "EA2"(w1085) -> ()
                n559 = local write "SI2"(w1080) -> ()
                n560 = local write "RO2"(w1081) -> ()
                n561 = local write "G2"(w1082) -> ()
                n562 = Not(x=w1106) -> (.not. x?=w1121:bool)
                n563 = Not(x=w1102) -> (.not. x?=w1124:bool)
                n564 = Not(x=w1101) -> (.not. x?=w1122:bool)
                n565 = Not(x=w1100) -> (.not. x?=w1123:bool)
                n566 = Not(x=w1105) -> (.not. x?=w1126:bool)
                n567 = Not(x=w1104) -> (.not. x?=w1125:bool)
                n568 = Not(x=w1103) -> (.not. x?=w1127:bool)
                n569 = property on="Acquisition Mode 2" class="Ring (strict)"("Blinking"=w1121) -> ()  [unwired: 2 in, 2 out]
                n570 = property on="Readout Rate 2" class="Ring (strict)"("Blinking"=w1124) -> ()  [unwired: 2 in, 2 out]
                n571 = property on="Vertical Shift Speed 2" class="Ring (strict)"("Blinking"=w1122) -> ()  [unwired: 2 in, 2 out]
                n572 = property on="CCD EM Mode 2" class="Ring (strict)"("Blinking"=w1123) -> ()  [unwired: 2 in, 2 out]
                n573 = property on="Trigger Mode 2" class="Ring (strict)"("Blinking"=w1126) -> ()  [unwired: 2 in, 2 out]
                n574 = property on="Read Mode 2" class="Ring (strict)"("Blinking"=w1125) -> ()  [unwired: 2 in, 2 out]
                n575 = property on="Pre-amplification Gain 2" class="Ring (strict)"("Blinking"=w1127) -> ()  [unwired: 2 in, 2 out]
                n576 = local write "Cameras Cluster"(w1153) -> ()
                n577 = Compound Arithmetic op=AND(w1106, w1105, w1104, w1103, w1102, w1101, w1100, w1113, w1112, w1111, w1110, w1109, w1108, w1107, w1120, w1119, w1118, w1117, w1116, w1115, w1114) -> (→"CCD checked 2":bool)
              }
              frame #17 {
                # "Carrega coluna do Channel 3"
                # "Aba:  Eng->Camera"
                n578 = Unbundle By Name(w1288) -> ("ChannelC_CCD"=w1220:T21, "CHC_Checked Params"=w1273:T22, "ChannelC_Status.connection"=w1213:bool)
                n579 = Unbundle By Name(w1273) -> ("ACQUISITION_MODE"=w1236:bool, "TRIGGER_MODE"=w1235:bool, "READ_MODE"=w1234:bool, "PREAMP"=w1233:bool, "READOUT_RATE"=w1232:bool, "VERTICAL_SHIFT_SPEED"=w1231:bool, "EM_MODE"=w1230:bool, "EM_GAIN"=w1244:bool, "SHUTTER_MODE"=w1243:bool, "SHUTTER_TTL"=w1241:bool, "SHUTTER_OPENING_TIME"=w1240:bool, "SHUTTER_CLOSING_TIME"=w1239:bool, "VBIN"=w1238:bool, "HBIN"=w1237:bool, "INITIAL_LINE"=w1251:bool, "INITIAL_COLUMN"=w1250:bool, "FINAL_LINE"=w1249:bool, "FINAL_COLUMN"=w1248:bool, "FRAME_TRANSFER"=w1247:bool, "VERTICAL_CLOCK_VOLTAGE"=w1246:bool, "AD_CHANNEL"=w1245:bool)
                n580 = case shown="True" w1213 {
                  tunnel: w1220 -> [_ w1296]
                  tunnel: [w1289 w1295] -> w1219
                  tunnel: [w1289 w1294] -> w1218
                  tunnel: [w1289 w1293] -> w1217
                  tunnel: [w1289 w1292] -> w1216
                  tunnel: [w1289 w1291] -> w1215
                  tunnel: [w1289 w1290] -> w1214
                  frame False {
                    w1289 = ""
                  }
                  frame True {
                    n581 = stacked-sequence "Atualizacao dos indicadores inferiores do CANAL C da tela principal" {
                      tunnel: w1296 -> [w1311 w1314 w1319 w1328 w1331 w1335]
                      tunnel: [w1297 _ _ _ _ _] -> w1295
                      tunnel: [_ w1312 _ _ _ _] -> w1294
                      tunnel: [_ _ w1317 _ _ _] -> w1293
                      tunnel: [_ _ _ w1322 _ _] -> w1292
                      tunnel: [_ _ _ _ w1329 _] -> w1291
                      tunnel: [_ _ _ _ _ w1332] -> w1290
                      frame #0 {
                        # "SubImage"
                        n582 = Unbundle By Name(w1311) -> ("INITIAL_LINE"=w1309:u16, "FINAL_LINE"=w1308:u16, "INITIAL_COLUMN"=w1307:u16, "FINAL_COLUMN"=w1306:u16)
                        n583 = Number To Decimal String(number=w1309) -> (decimal integer string=w1305:string)  [unwired: 1 in]
                        n584 = Number To Decimal String(number=w1308) -> (decimal integer string=w1303:string)  [unwired: 1 in]
                        n585 = Number To Decimal String(number=w1307) -> (decimal integer string=w1301:string)  [unwired: 1 in]
                        n586 = Number To Decimal String(number=w1306) -> (decimal integer string=w1299:string)  [unwired: 1 in]
                        n587 = Concatenate Strings("[", w1305, ":", w1303, ",", w1301, ":", w1299, "]") -> (w1297:string)
                      }
                      frame #1 {
                        # "Em Active"
                        n588 = Unbundle By Name(w1314) -> ("EM_MODE"=w1313:u8)
                        n589 = case shown="0, Default" w1313 {
                          tunnel: ["Electron M." ("EmActive1") "Convent." ("EmActive1")] -> w1312
                          frame 0, Default {
                          }
                          frame 1 {
                          }
                        }
                      }
                      frame #2 {
                        # "Pre Amp"
                        n590 = Unbundle By Name(w1319) -> ("PREAMP"=w1318:u8)
                        n591 = case shown="1" w1318 {
                          tunnel: ["Gain 1" ("EmActive1") "Gain 2" ("EmActive1")] -> w1317
                          frame 0, Default {
                          }
                          frame 1 {
                          }
                        }
                      }
                      frame #3 {
                        # "Binning"
                        n592 = Unbundle By Name(w1328) -> ("VBIN"=w1327:u16, "HBIN"=w1326:u16)
                        n593 = Number To Decimal String(number=w1326) -> (decimal integer string=w1323:string)  [unwired: 1 in]
                        n594 = Number To Decimal String(number=w1327) -> (decimal integer string=w1325:string)  [unwired: 1 in]
                        n595 = Concatenate Strings(w1325, "x", w1323) -> (w1322:string)
                      }
